vi "GetDTCConfig.vi"(0 "Server":string, 1 "Sequence Context In":refnum<k7>, 3 "Username":string, 5 "error in (no error)":errorcluster, 9 "ParamType":string, 11 "subMachine":string, 12 "MechID":string) -> (15 "error out":errorcluster)   [LabVIEW 2017]
uses:
  C:/Users/operator/Documents/DTC Map/Sensata.MES.Integration.ST.ParameterControl.dll
  Users/operator/Documents/DTC Map/Sensata.MES.Integration.ST.ParameterControl.dll
panel:
  out "GetParameterSetJSON":string
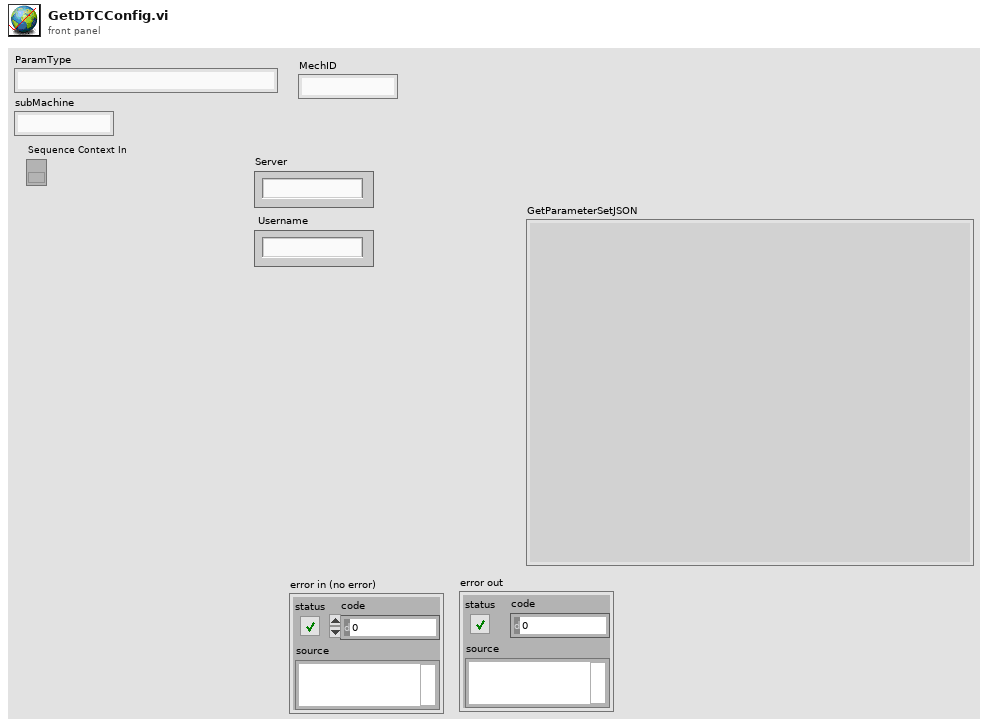
[diagram p1: front panel]
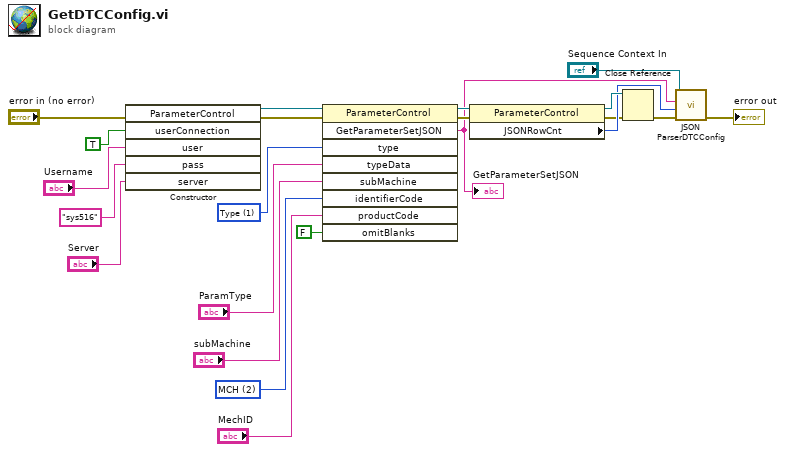
[diagram p0: block diagram]
diagram:
  w16 = 2 items=["BOM", "SMT", "MCH"] ("identifierCode")
  w19 = 1 items=["Process", "Type"] ("type")
  n1 = constructor class="ParameterControl"(error in="error in (no error)", "userConnection"=TRUE, "user"="Username", "pass"="sys516", "server"="Server") -> (reference out=w21:refnum<k24>, error out=w20:errorcluster)  [unwired: 2 in, 5 out]
  n2 = invoke class="ParameterControl" method="GetParameterSetJSON"(reference=w21, error in=w20, "type"=w19, "typeData"="ParamType", "subMachine"="subMachine", "identifierCode"=w16, "productCode"="MechID", "omitBlanks"=FALSE) -> (reference out=w13:refnum<k24>, error out=w12:errorcluster, "GetParameterSetJSON"=w9:string)  [unwired: 1 in, 6 out]
  "GetParameterSetJSON" <- w9
  n3 = property class="ParameterControl"(reference=w13, error in=w12) -> (reference out=w11:refnum<k24>, error out=w7:errorcluster, "JSONRowCnt"=w8:i32)
  n4 = Close Reference(reference=w11, error in (no error)=w7) -> (error out=w3:errorcluster)
  n5 = call "JSON ParserDTCConfig.vi"("Error In"=w3, "NumElements"=w8, "jsonin"=w9, "Sequence Context In"="Sequence Context In") -> ("error out"=→"error out":errorcluster)  [unwired: 7 in]
